vi "update delta t.vi"(8 "error in (no error)":errorcluster, 11 "Game Data in":T1) -> (0 "error out":errorcluster, 3 "Game Data out":T1)   [LabVIEW 2025]
uses:
  Game Data.ctl
  Bullet Data.ctl
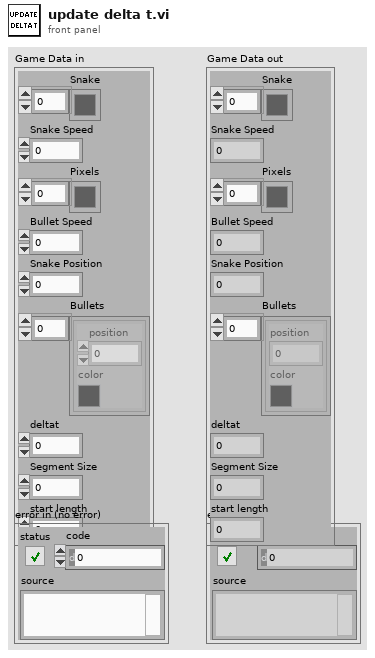
[diagram p1: front panel]
types:
  T1 = typedef "Game Data.ctl" = cluster{"Snake":u32[], "Snake Speed":dbl, "Pixels":u32[], "Bullet Speed":dbl, "Snake Position":dbl, "Bullets":T2[], "deltat":dbl, "Segment Size":dbl, "start length":u32}
  T2 = typedef "Bullet Data.ctl" = cluster{"position":dbl, "color":u32}
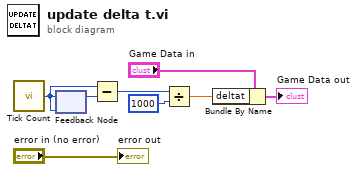
[diagram p0: block diagram]
diagram:
  n1 = call "Tick Count"() -> ("Tick Count(mSec)"=w4:u32)
  n2 = feedback-in #1(w4) -> ()
  n3 = feedback #1(w4) -> (w5:u32)
  n4 = Subtract(x=w4, y=w5) -> (x-y=w3:u32)
  n5 = Divide(x=w3, y=u32 1000) -> (x/y=w1:dbl)
  n6 = Bundle By Name(cluster="Game Data in", "deltat"=w1) -> (→"Game Data out":T1)
  "error out" <- "error in (no error)"
